vi "Begin.vi"(8 "error in":errorcluster) -> (0 "error out":errorcluster)   [LabVIEW 2019]
doc: "Called before other user functions, this VI is expected to open initial I/O refnums, load in file data, and do all program initialization. Notice that the <B>error out</B> terminal is simply used for data flow. Wiring it to other structures or subVIs ensures that this VI runs first."
uses:
  <vilib>/Rock Robotics/WPI/DriverStation/WPI_DriverStationRobotMode2.ctl
  <vilib>/Rock Robotics/WPI/Joystick/WPI_JoystickDeviceEnum.ctl
  <vilib>/Rock Robotics/SystemInterfaces/DIO/FPGA_DIOChannel.ctl
  <vilib>/Rock Robotics/WPI/Encoder/WPI_EncoderType.ctl
  <vilib>/Rock Robotics/WPI/ThirdParty/REV Robotics/SPARK MAX/Typedef/Spark MAX Motor Type.ctl
  <vilib>/Rock Robotics/WPI/ThirdParty/REV Robotics/SPARK MAX/Typedef/Spark MAX Idle Mode.ctl
  <vilib>/Rock Robotics/WPI/SafetyOutput/WPI_SafetyOutputConfigMenu.ctl
  Robot Global Data.vi
  <vilib>/Rock Robotics/WPI/Counter/WPI_CounterDigitalInputToDigitalSource.vi
  <vilib>/Rock Robotics/WPI/RobotDrive/WPI_RobotDriveOpen4MotorWithExistingMotors.vi
  <vilib>/Rock Robotics/Network Tables/NT Write String Array.vi
  <vilib>/Rock Robotics/WPI/ThirdParty/Phoenix-LabVIEW/Motor Controller/Controls/CTRE_Phoenix_MotorControl_ControlMode.ctl
  <vilib>/Rock Robotics/WPI/Solenoid/WPI_SolenoidChannel.ctl
  <vilib>/Rock Robotics/WPI/Solenoid/WPI_SolenoidOpenDouble.vi
  <vilib>/Rock Robotics/WPI/Switch/WPI_SwitchOpenLimit.vi
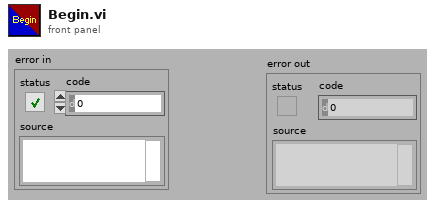
[diagram p1: front panel]
types:
  T1 = typedef "FPGA_DIOChannel.ctl" = enum8{"DIO 0", "DIO 1", "DIO 2", "DIO 3", "DIO 4", "DIO 5", "DIO 6", "DIO 7", "DIO 8", "DIO 9", "DIO MXP 0", "DIO MXP 1", "DIO MXP 2", "DIO MXP 3", "DIO MXP 4", "DIO MXP 5", "DIO MXP 6", "DIO MXP 7", "DIO MXP 8", "DIO MXP 9", "DIO MXP 10", "DIO MXP 11", "DIO MXP 12", "DIO MXP 13", "DIO MXP 14", "DIO MXP 15", "SPI Port CS1", "SPI Port CS2", "SPI Port CS3", "SPI Port MISO", "SPI Port MOSI", "Invalid"}
  T2 = typedef "CTRE_Phoenix_MotorControl_ControlMode.ctl" = u16
  T3 = typedef "WPI_SolenoidChannel.ctl" = enum8{"Solenoid 0", "Solenoid 1", "Solenoid 2", "Solenoid 3", "Solenoid 4", "Solenoid 5", "Solenoid 6", "Solenoid 7", "Invalid"}
  T4 = typedef "WPI_SafetyOutputConfigMenu.ctl" = enum16{"Enable", "Disable"}
  T5 = typedef "Spark MAX Idle Mode.ctl" = enum16{"Coast", "Brake"}
  T6 = typedef "Spark MAX Motor Type.ctl" = enum16{"Brushed", "Brushless"}
  T7 = typedef "WPI_EncoderType.ctl" = enum16{"1x", "2x", "4x"}
  T8 = typedef "WPI_JoystickDeviceEnum.ctl" = enum16{"USB 0", "USB 1", "USB 2", "USB 3", "USB 4", "USB 5"}
  T9 = typedef "WPI_DriverStationRobotMode2.ctl" = enum16{"Autonomous Disabled", "Autonomous Enabled", "Teleop Disabled", "Teleop Enabled", "Disconnected", "Finish", "Test Disabled", "Test Enabled", "Emergency Stopped"}
  T10 = typedef "WPI_MotorControlDeviceRef.ctl" = cluster{"DeviceStatus":errorcluster, "Type":T11, "PWM":cluster{"PWM Channel":T12, "DeadBand":T13}, "CAN":cluster{"Device Number":u8, "SetOutput VI Ref":variant, "GetOutput VI Ref":variant, "Enable VI Ref":variant, "Disable VI Ref":variant, "Data":variant}, "Invert":bool, "DIO PWM":cluster{"PWM \"Enable\" Channel":T12, "DIOChannel":T1, "PWM Rate":dbl}}
  T11 = typedef "WPI_MotorControlType.ctl" = enum16{"PWM", "CAN", "DIO PWM"}
  T12 = typedef "FPGA_DIOPWMChannel.ctl" = enum8{"PWM 0", "PWM 1", "PWM 2", "PWM 3", "PWM 4", "PWM 5", "PWM 6", "PWM 7", "PWM 8", "PWM 9", "PWM MXP 0", "PWM MXP 1", "PWM MXP 2", "PWM MXP 3", "PWM MXP 4", "PWM MXP 5", "PWM MXP 6", "PWM MXP 7", "PWM MXP 8", "PWM MXP 9", "Invalid"}
  T13 = typedef "WPI_PWMDeadband.ctl" = cluster{"Name":string, "maxPositivePwm":i32, "minPositivePwm":i32, "centerPwm":i32, "maxNegativePwm":i32, "minNegativePwm":i32, "angularRange":u16}
  T14 = typedef "WPI_JoystickDevRef.ctl" = cluster{"Device":T8}
  T15 = typedef "WPI_RobotDriveDevRef.ctl" = cluster{"DevStatus":errorcluster, "Motors[]":T10[], "Square Inputs":bool, "Max Output":dbl}
  T16 = typedef "WPI_SolenoidDevRef.ctl" = cluster{"DevStatus":errorcluster, "Pneumatics Control Module":u8, "Forward Solenoid Channel":T3, "Reverse Solenoid Channel":T3}
  T17 = typedef "WPI_DigitalInputDevRef.ctl" = cluster{"DevStatus":errorcluster, "DIO Channel":T1}
  T18 = typedef "FPGA_CounterEncoderSourceConvertionLVSourceType.ctl" = cluster{"DevStatus":errorcluster, "AnalogTriggerMode?":bool, "DigitalMode":cluster{"DIO Channel":T19}, "AnalogTriggerMode":cluster{"AnalogTriggerIndex":T20, "OutputType":T21}}
  T19 = typedef "FPGA_DIODigitalSourceChannel.ctl" = enum8{"DIO 0", "DIO 1", "DIO 2", "DIO 3", "DIO 4", "DIO 5", "DIO 6", "DIO 7", "DIO 8", "DIO 9", "DIO MXP 0", "DIO MXP 1", "DIO MXP 2", "DIO MXP 3", "DIO MXP 4", "DIO MXP 5", "DIO MXP 6", "DIO MXP 7", "DIO MXP 8", "DIO MXP 9", "DIO MXP 10", "DIO MXP 11", "DIO MXP 12", "DIO MXP 13", "DIO MXP 14", "DIO MXP 15", "SPI Port CS1", "SPI Port CS2", "SPI Port CS3", "SPI Port MISO", "SPI Port MOSI", "Disabled"}
  T20 = typedef "FPGA_AnalogTriggerIndex.ctl" = enum8{"Trig 0", "Trig 1", "Trig 2", "Trig 3", "Trig 4", "Trig 5", "Trig 6", "Trig 7", "Invalid"}
  T21 = typedef "FPGA_AnalogTriggerOutType.ctl" = enum16{"InWindow", "TriggerState", "Rising", "Falling"}
  T22 = typedef "WPI_EncoderDevRef.ctl" = cluster{"DevStatus":errorcluster, "EncoderIndex":T23, "CounterIndex":T24, "DistancePerCount":dbl, "Decoding Type":T7}
  T23 = typedef "FPGA_EncoderIdx.ctl" = enum8{"Enc 0", "Enc 1", "Enc 2", "Enc 3", "Enc 4", "Enc 5", "Enc 6", "Enc 7", "Invalid"}
  T24 = typedef "FPGA_CounterCtrSystemIndex.ctl" = enum8{"Ctr 0", "Ctr 1", "Ctr 2", "Ctr 3", "Ctr 4", "Ctr 5", "Ctr 6", "Ctr 7", "Invalid"}
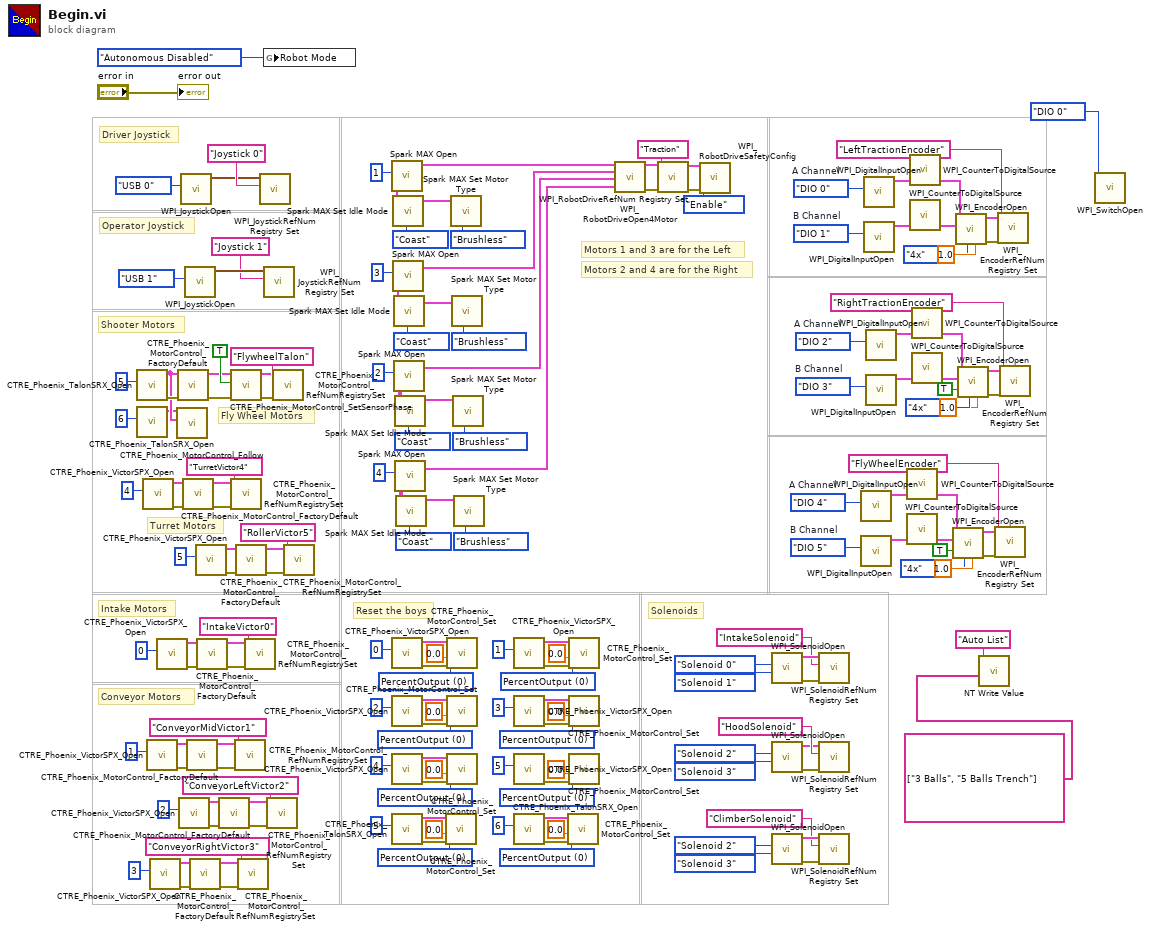
[diagram p0: block diagram]
diagram:
  w2 = T2 0 items=["PercentOutput"=0, "Position"=1, "Velocity"=2, "Current"=3, "Follower"=5, "MotionProfile"=6, "MotionMagic"=7, "MotionMagicArc"=8, "MotionProfileArc"=10, "Disabled"=15] ("Control Mode")
  w26 = T2 0 items=["PercentOutput"=0, "Position"=1, "Velocity"=2, "Current"=3, "Follower"=5, "MotionProfile"=6, "MotionMagic"=7, "MotionMagicArc"=8, "MotionProfileArc"=10, "Disabled"=15] ("Control Mode")
  w32 = T2 0 items=["PercentOutput"=0, "Position"=1, "Velocity"=2, "Current"=3, "Follower"=5, "MotionProfile"=6, "MotionMagic"=7, "MotionMagicArc"=8, "MotionProfileArc"=10, "Disabled"=15] ("Control Mode")
  w31 = T2 0 items=["PercentOutput"=0, "Position"=1, "Velocity"=2, "Current"=3, "Follower"=5, "MotionProfile"=6, "MotionMagic"=7, "MotionMagicArc"=8, "MotionProfileArc"=10, "Disabled"=15] ("Control Mode")
  w41 = T2 0 items=["PercentOutput"=0, "Position"=1, "Velocity"=2, "Current"=3, "Follower"=5, "MotionProfile"=6, "MotionMagic"=7, "MotionMagicArc"=8, "MotionProfileArc"=10, "Disabled"=15] ("Control Mode")
  w42 = T2 0 items=["PercentOutput"=0, "Position"=1, "Velocity"=2, "Current"=3, "Follower"=5, "MotionProfile"=6, "MotionMagic"=7, "MotionMagicArc"=8, "MotionProfileArc"=10, "Disabled"=15] ("Control Mode")
  w51 = T2 0 items=["PercentOutput"=0, "Position"=1, "Velocity"=2, "Current"=3, "Follower"=5, "MotionProfile"=6, "MotionMagic"=7, "MotionMagicArc"=8, "MotionProfileArc"=10, "Disabled"=15] ("Control Mode")
  w52 = T2 0 items=["PercentOutput"=0, "Position"=1, "Velocity"=2, "Current"=3, "Follower"=5, "MotionProfile"=6, "MotionMagic"=7, "MotionMagicArc"=8, "MotionProfileArc"=10, "Disabled"=15] ("Control Mode")
  w136 = FPGA_DIOChannel."DIO 5"  # B Channel
  w135 = FPGA_DIOChannel."DIO 4"  # A Channel
  w139 = FPGA_DIOChannel."DIO 3"  # B Channel
  w140 = FPGA_DIOChannel."DIO 2"  # A Channel
  w160 = FPGA_DIOChannel."DIO 1"  # B Channel
  w159 = FPGA_DIOChannel."DIO 0"  # A Channel
  # "Solenoids"
  # "Reset the boys"
  # "Conveyor Motors"
  # "Intake Motors"
  # "Turret Motors"
  # "Fly Wheel Motors"
  # "Shooter Motors"
  # "Motors 2 and 4 are for the Right"
  # "Motors 1 and 3 are for the Left"
  # "Operator Joystick"
  # "Driver Joystick"
  n1 = call <vilib>:"CTRE_Phoenix_TalonSRX_Open.vi"("Device Number"=u8 5) -> ("error out"=w96:errorcluster, "CAN Talon SRX Ref"=w95:T10)  [unwired: 9 in]
  n2 = call <vilib>:"CTRE_Phoenix_TalonSRX_Open.vi"("Device Number"=u8 6) -> ("CAN Talon SRX Ref"=w58:T10)  [unwired: 9 in, 1 out]
  n3 = call <vilib>:"CTRE_Phoenix_VictorSPX_Open.vi"("Device Number"=u8 4) -> ("error out"=w70:errorcluster, "CAN Talon SRX Ref"=w69:T10)  [unwired: 9 in]
  n4 = call <vilib>:"CTRE_Phoenix_VictorSPX_Open.vi"("Device Number"=u8 1) -> ("error out"=w83:errorcluster, "CAN Talon SRX Ref"=w84:T10)  [unwired: 9 in]
  n5 = call <vilib>:"CTRE_Phoenix_VictorSPX_Open.vi"("Device Number"=u8 3) -> ("error out"=w71:errorcluster, "CAN Talon SRX Ref"=w72:T10)  [unwired: 9 in]
  n6 = call <vilib>:"CTRE_Phoenix_VictorSPX_Open.vi"("Device Number"=u8 0) -> ("error out"=w94:errorcluster, "CAN Talon SRX Ref"=w93:T10)  [unwired: 9 in]
  n7 = call <vilib>:"CTRE_Phoenix_MotorControl_Follow.vi"("Master Controller to Follow"=w95, "PhoenixMotorControlDevRef"=w58) -> ()  [unwired: 8 in, 2 out]
  n8 = call <vilib>:"CTRE_Phoenix_MotorControl_FactoryDefault.vi"("error in"=w96, "PhoenixMotorControlDevRef"=w95) -> ("error out"=w99:errorcluster, "PhoenixMotorControlDevRef"=w100:T10)  [unwired: 8 in]
  n9 = call <vilib>:"CTRE_Phoenix_VictorSPX_Open.vi"("Device Number"=u8 2) -> ("error out"=w82:errorcluster, "CAN Talon SRX Ref"=w81:T10)  [unwired: 9 in]
  n10 = call <vilib>:"WPI_JoystickOpen.vi"("JoystickDevice"=WPI_JoystickDeviceEnum."USB 0") -> ("JoystickDevRef"=w167:T14)  [unwired: 10 in]
  n11 = call <vilib>:"CTRE_Phoenix_MotorControl_FactoryDefault.vi"("error in"=w70, "PhoenixMotorControlDevRef"=w69) -> ("error out"=w68:errorcluster, "PhoenixMotorControlDevRef"=w66:T10)  [unwired: 8 in]
  n12 = call <vilib>:"WPI_JoystickOpen.vi"("JoystickDevice"=WPI_JoystickDeviceEnum."USB 1") -> ("JoystickDevRef"=w162:T14)  [unwired: 10 in]
  n13 = call <vilib>:"CTRE_Phoenix_MotorControl_FactoryDefault.vi"("error in"=w83, "PhoenixMotorControlDevRef"=w84) -> ("error out"=w85:errorcluster, "PhoenixMotorControlDevRef"=w86:T10)  [unwired: 8 in]
  n14 = call <vilib>:"CTRE_Phoenix_MotorControl_FactoryDefault.vi"("error in"=w71, "PhoenixMotorControlDevRef"=w72) -> ("error out"=w73:errorcluster, "PhoenixMotorControlDevRef"=w74:T10)  [unwired: 8 in]
  n15 = call <vilib>:"CTRE_Phoenix_VictorSPX_Open.vi"("Device Number"=u8 5) -> ("error out"=w59:errorcluster, "CAN Talon SRX Ref"=w60:T10)  [unwired: 9 in]
  n16 = call <vilib>:"CTRE_Phoenix_MotorControl_FactoryDefault.vi"("error in"=w94, "PhoenixMotorControlDevRef"=w93) -> ("error out"=w92:errorcluster, "PhoenixMotorControlDevRef"=w91:T10)  [unwired: 8 in]
  n17 = call <vilib>:"CTRE_Phoenix_MotorControl_FactoryDefault.vi"("error in"=w82, "PhoenixMotorControlDevRef"=w81) -> ("error out"=w80:errorcluster, "PhoenixMotorControlDevRef"=w79:T10)  [unwired: 8 in]
  n18 = call <vilib>:"CTRE_Phoenix_MotorControl_SetSensorPhase.vi"("error in (no error)"=w99, "PhaseSensor"=TRUE, "PhoenixMotorControlDevRef"=w100) -> ("error out"=w97:errorcluster, "PhoenixMotorControlDevRef"=w98:T10)  [unwired: 7 in]
  n19 = call <vilib>:"CTRE_Phoenix_MotorControl_RefNumRegistrySet.vi"("error in (no error)"=w68, "refnum name"="TurretVictor4", "PhoenixMotorControlDevRef"=w66) -> ()  [unwired: 7 in, 2 out]
  n20 = call <vilib>:"CTRE_Phoenix_MotorControl_RefNumRegistrySet.vi"("error in (no error)"=w85, "refnum name"="ConveyorMidVictor1", "PhoenixMotorControlDevRef"=w86) -> ()  [unwired: 7 in, 2 out]
  n21 = call <vilib>:"CTRE_Phoenix_MotorControl_FactoryDefault.vi"("error in"=w59, "PhoenixMotorControlDevRef"=w60) -> ("error out"=w61:errorcluster, "PhoenixMotorControlDevRef"=w63:T10)  [unwired: 8 in]
  n22 = call <vilib>:"CTRE_Phoenix_MotorControl_RefNumRegistrySet.vi"("error in (no error)"=w73, "refnum name"="ConveyorRightVictor3", "PhoenixMotorControlDevRef"=w74) -> ()  [unwired: 7 in, 2 out]
  n23 = call <vilib>:"CTRE_Phoenix_MotorControl_RefNumRegistrySet.vi"("error in (no error)"=w92, "refnum name"="IntakeVictor0", "PhoenixMotorControlDevRef"=w91) -> ()  [unwired: 7 in, 2 out]
  n24 = call <vilib>:"WPI_JoystickRefNum Registry Set.vi"("refnum name"="Joystick 0", "JoystickDevRef"=w167) -> ()  [unwired: 8 in, 2 out]
  n25 = global write "Robot Global Data.vi" "Robot Mode"(WPI_DriverStationRobotMode2."Autonomous Disabled" ("Robot Mode")) -> ()
  n26 = call <vilib>:"WPI_JoystickRefNum Registry Set.vi"("refnum name"="Joystick 1", "JoystickDevRef"=w162) -> ()  [unwired: 8 in, 2 out]
  n27 = call <vilib>:"CTRE_Phoenix_MotorControl_RefNumRegistrySet.vi"("error in (no error)"=w80, "refnum name"="ConveyorLeftVictor2", "PhoenixMotorControlDevRef"=w79) -> ()  [unwired: 7 in, 2 out]
  n28 = call <vilib>:"CTRE_Phoenix_MotorControl_RefNumRegistrySet.vi"("error in (no error)"=w97, "refnum name"="FlywheelTalon", "PhoenixMotorControlDevRef"=w98) -> ()  [unwired: 7 in, 2 out]
  n29 = call <vilib>:"CTRE_Phoenix_MotorControl_RefNumRegistrySet.vi"("error in (no error)"=w61, "refnum name"="RollerVictor5", "PhoenixMotorControlDevRef"=w63) -> ()  [unwired: 7 in, 2 out]
  n30 = call <vilib>:"Spark MAX Open.vi"("Device Number"=u8 1) -> ("MotorControlDeviceRef"=w122:T10)  [unwired: 9 in, 1 out]
  n31 = call <vilib>:"CTRE_Phoenix_VictorSPX_Open.vi"("Device Number"=u8 0) -> ("error out"=w46:errorcluster, "CAN Talon SRX Ref"=w45:T10)  [unwired: 9 in]
  n32 = call <vilib>:"CTRE_Phoenix_VictorSPX_Open.vi"("Device Number"=u8 2) -> ("error out"=w37:errorcluster, "CAN Talon SRX Ref"=w38:T10)  [unwired: 9 in]
  n33 = call <vilib>:"CTRE_Phoenix_VictorSPX_Open.vi"("Device Number"=u8 4) -> ("error out"=w22:errorcluster, "CAN Talon SRX Ref"=w23:T10)  [unwired: 9 in]
  n34 = call <vilib>:"CTRE_Phoenix_TalonSRX_Open.vi"("Device Number"=u8 5) -> ("error out"=w56:errorcluster, "CAN Talon SRX Ref"=w55:T10)  [unwired: 9 in]
  n35 = call <vilib>:"Spark MAX Set Idle Mode.vi"("Idle Mode"=Spark_MAX_Idle_Mode."Coast", "MotorControlDeviceRef in"=w122) -> ()  [unwired: 8 in, 2 out]
  n36 = call <vilib>:"Spark MAX Open.vi"("Device Number"=u8 3) -> ("MotorControlDeviceRef"=w118:T10)  [unwired: 9 in, 1 out]
  n37 = call <vilib>:"Spark MAX Set Idle Mode.vi"("Idle Mode"=Spark_MAX_Idle_Mode."Coast", "MotorControlDeviceRef in"=w118) -> ()  [unwired: 8 in, 2 out]
  n38 = call <vilib>:"Spark MAX Open.vi"("Device Number"=u8 2) -> ("MotorControlDeviceRef"=w114:T10)  [unwired: 9 in, 1 out]
  n39 = call <vilib>:"Spark MAX Set Idle Mode.vi"("Idle Mode"=Spark_MAX_Idle_Mode."Coast", "MotorControlDeviceRef in"=w114) -> ()  [unwired: 8 in, 2 out]
  n40 = call <vilib>:"Spark MAX Open.vi"("Device Number"=u8 4) -> ("MotorControlDeviceRef"=w110:T10)  [unwired: 9 in, 1 out]
  n41 = call <vilib>:"Spark MAX Set Idle Mode.vi"("Idle Mode"=Spark_MAX_Idle_Mode."Coast", "MotorControlDeviceRef in"=w110) -> ()  [unwired: 8 in, 2 out]
  n42 = call <vilib>:"CTRE_Phoenix_MotorControl_Set.vi"("error in (no error)"=w56, "Output"=0.0, "Control Mode"=w52, "PhoenixMotorControlDevRef"=w55) -> ()  [unwired: 6 in, 2 out]
  n43 = call <vilib>:"CTRE_Phoenix_MotorControl_Set.vi"("error in (no error)"=w46, "Output"=0.0, "Control Mode"=w42, "PhoenixMotorControlDevRef"=w45) -> ()  [unwired: 6 in, 2 out]
  n44 = call <vilib>:"CTRE_Phoenix_MotorControl_Set.vi"("error in (no error)"=w37, "Output"=0.0, "Control Mode"=w41, "PhoenixMotorControlDevRef"=w38) -> ()  [unwired: 6 in, 2 out]
  n45 = call <vilib>:"CTRE_Phoenix_MotorControl_Set.vi"("error in (no error)"=w22, "Output"=0.0, "Control Mode"=w26, "PhoenixMotorControlDevRef"=w23) -> ()  [unwired: 6 in, 2 out]
  n46 = call <vilib>:"Spark MAX Set Motor Type.vi"("Motor Type"=Spark_MAX_Motor_Type."Brushless", "MotorControlDevRef"=w122) -> ()  [unwired: 8 in, 2 out]
  n47 = call <vilib>:"Spark MAX Set Motor Type.vi"("Motor Type"=Spark_MAX_Motor_Type."Brushless", "MotorControlDevRef"=w118) -> ()  [unwired: 8 in, 2 out]
  n48 = call <vilib>:"Spark MAX Set Motor Type.vi"("Motor Type"=Spark_MAX_Motor_Type."Brushless", "MotorControlDevRef"=w114) -> ()  [unwired: 8 in, 2 out]
  n49 = call <vilib>:"Spark MAX Set Motor Type.vi"("Motor Type"=Spark_MAX_Motor_Type."Brushless", "MotorControlDevRef"=w110) -> ()  [unwired: 8 in, 2 out]
  n50 = call <vilib>:"CTRE_Phoenix_VictorSPX_Open.vi"("Device Number"=u8 1) -> ("error out"=w27:errorcluster, "CAN Talon SRX Ref"=w28:T10)  [unwired: 9 in]
  n51 = call <vilib>:"CTRE_Phoenix_VictorSPX_Open.vi"("Device Number"=u8 3) -> ("error out"=w36:errorcluster, "CAN Talon SRX Ref"=w35:T10)  [unwired: 9 in]
  n52 = call <vilib>:"CTRE_Phoenix_VictorSPX_Open.vi"("Device Number"=u8 5) -> ("error out"=w5:errorcluster)  [unwired: 9 in, 1 out]
  n53 = call <vilib>:"CTRE_Phoenix_TalonSRX_Open.vi"("Device Number"=u8 6) -> ("error out"=w47:errorcluster, "CAN Talon SRX Ref"=w48:T10)  [unwired: 9 in]
  n54 = call <vilib>:"CTRE_Phoenix_MotorControl_Set.vi"("error in (no error)"=w47, "Output"=0.0, "Control Mode"=w51, "PhoenixMotorControlDevRef"=w48) -> ()  [unwired: 6 in, 2 out]
  n55 = call <vilib>:"CTRE_Phoenix_MotorControl_Set.vi"("error in (no error)"=w27, "Output"=0.0, "Control Mode"=w31, "PhoenixMotorControlDevRef"=w28) -> ()  [unwired: 6 in, 2 out]
  n56 = call <vilib>:"CTRE_Phoenix_MotorControl_Set.vi"("error in (no error)"=w36, "Output"=0.0, "Control Mode"=w32, "PhoenixMotorControlDevRef"=w35) -> ()  [unwired: 6 in, 2 out]
  n57 = call <vilib>:"CTRE_Phoenix_MotorControl_Set.vi"("error in (no error)"=w5, "Output"=0.0, "Control Mode"=w2) -> ()  [unwired: 7 in, 2 out]
  n58 = call-poly <vilib>:"WPI_RobotDriveOpen4Motor.vi"("Rear Left Motor Dev Ref"=w122, "Rear Right Motor Dev Ref"=w118, "Front Left Motor Dev Ref"=w114, "Front Right Motor Dev Ref"=w110) -> ("RobotDriveDevRef"=w108:T15, "error out"=w109:errorcluster)  [unwired: 10 in]
  n59 = call <vilib>:"WPI_RobotDriveRefNum Registry Set.vi"("error in (no error)"=w109, "refnum name"="Traction", "RobotDriveDevRef"=w108) -> ("error out"=w106:errorcluster, "RobotDriveDevRef"=w105:T15)  [unwired: 7 in]
  n60 = call <vilib>:"WPI_RobotDriveSafetyConfig.vi"("error in (no error)"=w106, "mode"=WPI_SafetyOutputConfigMenu."Enable", "RobotDriveDevRef"=w105) -> ()  [unwired: 7 in, 2 out]
  n61 = call-poly <vilib>:"WPI_SolenoidOpen.vi"("Reverse Solenoid Channel"=WPI_SolenoidChannel."Solenoid 1", "Forward Solenoid Channel"=WPI_SolenoidChannel."Solenoid 0") -> ("error out"=w21:errorcluster, "SolenoidDevRef"=w20:T16)  [unwired: 8 in]
  n62 = call-poly <vilib>:"WPI_SolenoidOpen.vi"("Reverse Solenoid Channel"=WPI_SolenoidChannel."Solenoid 3", "Forward Solenoid Channel"=WPI_SolenoidChannel."Solenoid 2") -> ("error out"=w12:errorcluster, "SolenoidDevRef"=w13:T16)  [unwired: 8 in]
  n63 = call-poly <vilib>:"WPI_SolenoidOpen.vi"("Reverse Solenoid Channel"=WPI_SolenoidChannel."Solenoid 3", "Forward Solenoid Channel"=WPI_SolenoidChannel."Solenoid 2") -> ("error out"=w11:errorcluster, "SolenoidDevRef"=w10:T16)  [unwired: 8 in]
  n64 = call <vilib>:"WPI_SolenoidRefNum Registry Set.vi"("error in (no error)"=w21, "refnum name"="IntakeSolenoid", "SolenoidDevRef"=w20) -> ()  [unwired: 7 in, 2 out]
  n65 = call <vilib>:"WPI_SolenoidRefNum Registry Set.vi"("error in (no error)"=w12, "refnum name"="HoodSolenoid", "SolenoidDevRef"=w13) -> ()  [unwired: 7 in, 2 out]
  n66 = call <vilib>:"WPI_SolenoidRefNum Registry Set.vi"("error in (no error)"=w11, "refnum name"="ClimberSolenoid", "SolenoidDevRef"=w10) -> ()  [unwired: 7 in, 2 out]
  n67 = call <vilib>:"WPI_DigitalInputOpen.vi"("DIO Channel"=w135) -> ("DigitalInputDevRef"=w132:T17)  [unwired: 1 in, 9 out]
  n68 = call <vilib>:"WPI_DigitalInputOpen.vi"("DIO Channel"=w136) -> ("DigitalInputDevRef"=w133:T17)  [unwired: 1 in, 9 out]
  n69 = call <vilib>:"WPI_DigitalInputOpen.vi"("DIO Channel"=w159) -> ("DigitalInputDevRef"=w156:T17)  [unwired: 1 in, 9 out]
  n70 = call <vilib>:"WPI_DigitalInputOpen.vi"("DIO Channel"=w160) -> ("DigitalInputDevRef"=w157:T17)  [unwired: 1 in, 9 out]
  n71 = call <vilib>:"WPI_DigitalInputOpen.vi"("DIO Channel"=w140) -> ("DigitalInputDevRef"=w143:T17)  [unwired: 1 in, 9 out]
  n72 = call <vilib>:"WPI_DigitalInputOpen.vi"("DIO Channel"=w139) -> ("DigitalInputDevRef"=w142:T17)  [unwired: 1 in, 9 out]
  n73 = call-poly <vilib>:"WPI_CounterToDigitalSource.vi"("DigitalInputDevRef"=w132) -> ("Digital Source"=w131:T18)  [unwired: 6 out]
  n74 = call-poly <vilib>:"WPI_CounterToDigitalSource.vi"("DigitalInputDevRef"=w133) -> ("Digital Source"=w134:T18)  [unwired: 6 out]
  n75 = call-poly <vilib>:"WPI_CounterToDigitalSource.vi"("DigitalInputDevRef"=w156) -> ("Digital Source"=w155:T18)  [unwired: 6 out]
  n76 = call-poly <vilib>:"WPI_CounterToDigitalSource.vi"("DigitalInputDevRef"=w157) -> ("Digital Source"=w158:T18)  [unwired: 6 out]
  n77 = call-poly <vilib>:"WPI_CounterToDigitalSource.vi"("DigitalInputDevRef"=w143) -> ("Digital Source"=w144:T18)  [unwired: 6 out]
  n78 = call-poly <vilib>:"WPI_CounterToDigitalSource.vi"("DigitalInputDevRef"=w142) -> ("Digital Source"=w141:T18)  [unwired: 6 out]
  n79 = call <vilib>:"WPI_EncoderOpen.vi"("DistancePerCount"=1.0, "Decoding Type"=WPI_EncoderType."4x", "Invert Direction (False)"=TRUE, "BSource"=w134, "ASource"=w131) -> ("error out"=w128:errorcluster, "EncoderDevRef"=w127:T22)  [unwired: 3 in, 2 out]
  n80 = call <vilib>:"WPI_EncoderOpen.vi"("DistancePerCount"=1.0, "Decoding Type"=WPI_EncoderType."4x", "BSource"=w158, "ASource"=w155) -> ("error out"=w152:errorcluster, "EncoderDevRef"=w151:T22)  [unwired: 4 in, 2 out]
  n81 = call <vilib>:"WPI_EncoderOpen.vi"("DistancePerCount"=1.0, "Decoding Type"=WPI_EncoderType."4x", "Invert Direction (False)"=TRUE, "BSource"=w141, "ASource"=w144) -> ("error out"=w147:errorcluster, "EncoderDevRef"=w148:T22)  [unwired: 3 in, 2 out]
  n82 = call-poly <vilib>:"NT Write Value.vi"("String Array"=string[] ["3 Balls", "5 Balls Trench"], "Name"="Auto List") -> ()  [unwired: 9 in, 1 out]
  n83 = call <vilib>:"WPI_EncoderRefNum Registry Set.vi"("error in (no error)"=w128, "refnum name"="FlyWheelEncoder", "EncoderDevRef"=w127) -> ()  [unwired: 7 in, 2 out]
  n84 = call <vilib>:"WPI_EncoderRefNum Registry Set.vi"("error in (no error)"=w152, "refnum name"="LeftTractionEncoder", "EncoderDevRef"=w151) -> ()  [unwired: 7 in, 2 out]
  n85 = call <vilib>:"WPI_EncoderRefNum Registry Set.vi"("error in (no error)"=w147, "refnum name"="RightTractionEncoder", "EncoderDevRef"=w148) -> ()  [unwired: 7 in, 2 out]
  n86 = call-poly <vilib>:"WPI_SwitchOpen.vi"("DIO Channel"=FPGA_DIOChannel."DIO 0") -> ()  [unwired: 9 in, 2 out]
  "error out" <- "error in"
